vi "GetConfigDirectory.vi"(8 "error in":errorcluster, 11 "Config File Directory":path) -> (0 "error out":errorcluster, 3 "config file directory out":path)   [LabVIEW 2014]
uses:
  <vilib>/Utility/sysdir.llb/System Directory Type.ctl
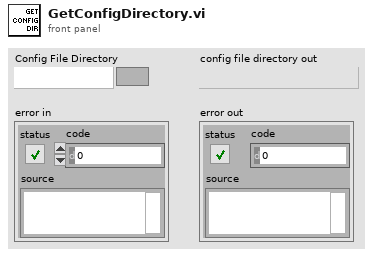
[diagram p1: front panel]
types:
  T1 = typedef "System Directory Type.ctl" = i32
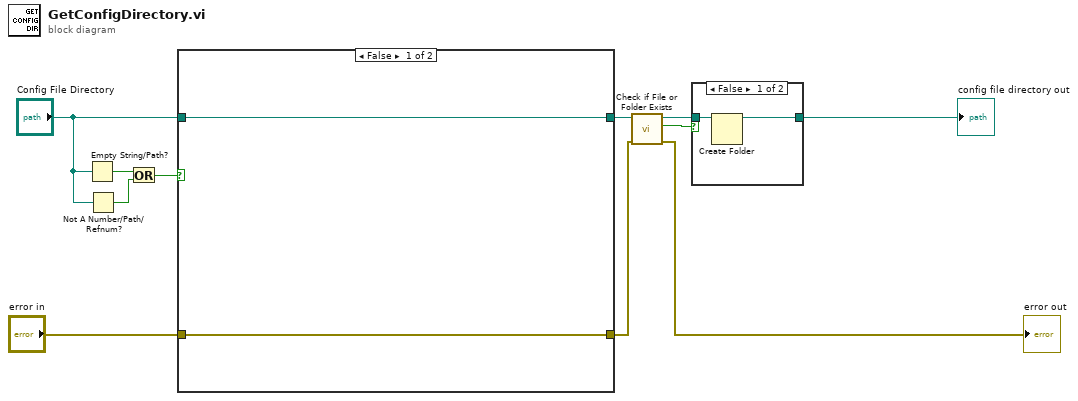
[diagram p0: block diagram]
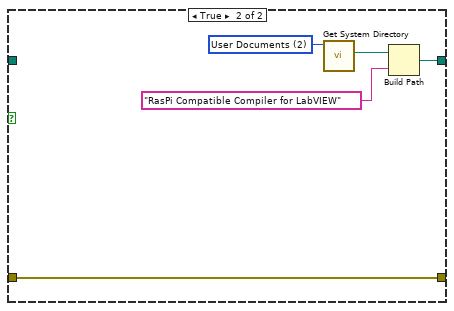
[diagram p2: hidden frame]
diagram:
  n1 = Empty String/Path?(string/path="Config File Directory") -> (empty?=w7:bool)
  n2 = Not A Number/Path/Refnum?(number/path/refnum="Config File Directory") -> (NaN/Path/Refnum?=w8:bool)
  n3 = Or(x=w7, y=w8) -> (x .or. y?=w5:bool)
  n4 = case shown="False" w5 {
    tunnel: [w13 w18] -> w2
    tunnel: "Config File Directory" -> [w13 _]
    tunnel: "error in" -> [w12 w14]
    tunnel: [w12 w14] -> w10
    frame False {
    }
    frame True {
      w17 = T1 2 items=["User Home"=0, "User Desktop"=1, "User Documents"=2, "User Application Data"=3, "User Preferences"=4, "User Temporary"=5, "Public Documents"=6, "Public Application Data"=7, "Public Preferences"=8, "Public Cache"=13, "System Core Libraries"=9, "System Installed Libraries"=10, "Application Files"=11, "Boot Volume Root"=12] ("system directory type")
      n5 = call <vilib>:"Get System Directory.vi"("system directory type"=w17) -> ("system directory"=w16:path)  [unwired: 10 in]
      n6 = Build Path(base path=w16, name or relative path="RasPi Compatible Compiler for LabVIEW") -> (appended path=w18:path)
    }
  }
  n7 = call <vilib>:"Check if File or Folder Exists.vi"("error in (no error)"=w10, "path"=w2) -> ("error out"=→"error out":errorcluster, "file or folder exists?"=w3:bool, "dup path"=w4:path)  [unwired: 7 in]
  n8 = case shown="False" w3 {
    tunnel: [w20 w21] -> w1
    tunnel: w4 -> [w19 w21]
    frame False {
      n9 = Create Folder(path (use dialog)=w19) -> (created path=w20:path)  [unwired: 2 in, 2 out]
    }
    frame True {
    }
  }
  "config file directory out" <- w1
